vi "Load.vi"(8 "error in (no error)":errorcluster) -> (0 "error out":errorcluster)   [LabVIEW 2020, in "WebServiceImporter.lvlib" / "Main Panel.lvlib" / "Progress.lvlib"]
uses:
  <vilib>/Platform/WebService/Main Panel/Pages/Progress/Progress.lvlib
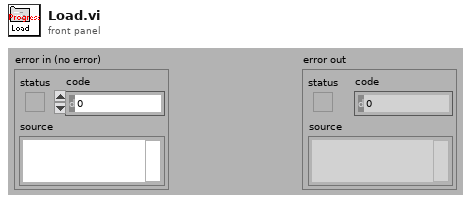
[diagram p1: front panel]
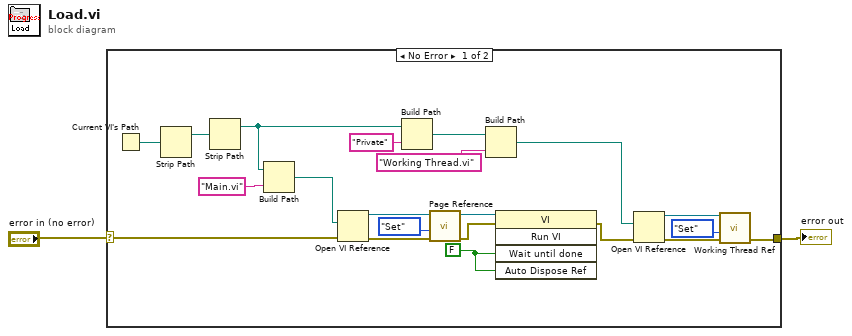
[diagram p0: block diagram]
diagram:
  n1 = case shown="No Error" "error in (no error)" {
    selector: "error in (no error)" -> [w17 w23]
    tunnel: [w9 w23] -> w1
    frame No Error {
      w3 = FALSE
      n2 = Current VI's Path() -> (path=w22:path)
      n3 = Strip Path(path=w22) -> (stripped path=w21:path)  [unwired: 1 out]
      n4 = Strip Path(path=w21) -> (stripped path=w16:path)  [unwired: 1 out]
      n5 = Build Path(base path=w16, name or relative path="Main.vi") -> (appended path=w19:path)
      n6 = Open VI Reference(vi path=w19, error in (no error)=w17) -> (vi reference=w18:refnum<vi>, error out=w8:errorcluster)  [unwired: 4 in]
      n7 = Build Path(base path=w16, name or relative path="Private") -> (appended path=w14:path)
      n8 = call <vilib>:"Page Reference.vi"("error in (no error)"=w8, "Operation"=enum16{"Get", "Set"}."Set", "VI Refnum"=w18) -> ("error out"=w5:errorcluster, "VI Refnum (out)"=w6:refnum<vi>)  [unwired: 7 in]
      n9 = Build Path(base path=w14, name or relative path="Working Thread.vi") -> (appended path=w12:path)
      n10 = invoke class="VI" method="Run VI"(reference=w6, error in=w5, "Wait until done"=w3, "Auto Dispose Ref"=w3) -> (error out=w4:errorcluster)  [unwired: 1 in, 4 out]
      n11 = Open VI Reference(vi path=w12, error in (no error)=w4) -> (vi reference=w10:refnum<vi>, error out=w9:errorcluster)  [unwired: 4 in]
      n12 = call <vilib>:"Working Thread Ref.vi"("Operation"=enum16{"Get", "Set"}."Set", "VI Refnum"=w10) -> ()  [unwired: 8 in, 2 out]
    }
    frame Error {
    }
  }
  "error out" <- w1
